vi "test_RS-xxx Write.vi"(8 "error in (no error)":errorcluster, 11 "TestCase in":refnum<class "Instrument Addon Serial Protocols Unit Tests.lvclass">) -> (0 "error out":errorcluster, 3 "TestCase out":refnum<class "Instrument Addon Serial Protocols Unit Tests.lvclass">)   [LabVIEW 2018, in "Instrument Addon Serial Protocols Unit Tests.lvclass"]
uses:
  Instrument Addon Serial Protocols Unit Tests.lvclass
  Listener/Listener.lvclass
  Listener/ListenerClassControls/Operation.ctl
  RS-xxx/RS-xxx.lvclass
  C:/Dev/niveristand-instrument-addon-classes/Source/Protocols/Protocol Parent/Protocol Parent.lvclass
  <vilib>/Platform/TimedLoop/XDataNode/timing_clust.ctl
  <vilib>/Platform/TimedLoop/XDataNode/nitl_modes.ctl
  <vilib>/Platform/TimedLoop/XDataNode/wakeup.ctl
  RS-xxx/RS-xxx.lvclass/RS-xxx.ctl
  <vilib>/platform/TimedLoop/XDataNode/XDataNode.xnode
  <vilib>/addons/_JKI Toolkits/VI Tester/TestCase.llb/TestCase.lvclass
  <vilib>/Platform/TimedLoop/XDataNode/XDNodeRunTimeDep.lvlib
  C:/Program Files (x86)/National Instruments/LabVIEW 2018/vi.lib/addons/_JKI Toolkits/VI Tester/TestCase.llb/TestCase.lvclass
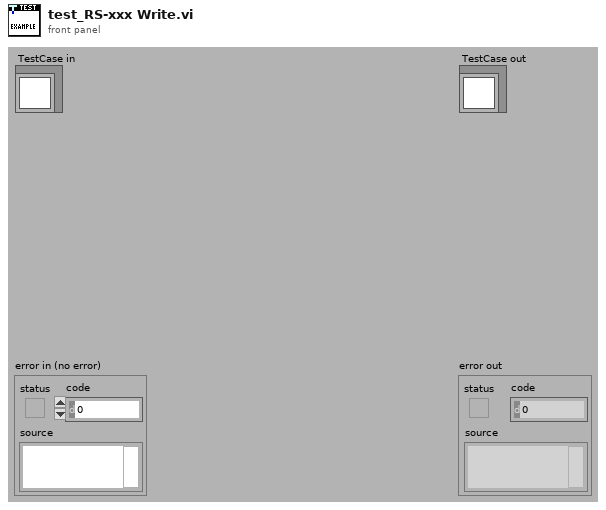
[diagram p1: front panel]
types:
  T1 = typedef "Listener.lvclass/Operation.ctl" = enum16{"Read", "Write"}
  T2 = typedef "XDNodeRunTimeDep.lvlib/timing_clust.ctl" = cluster{"Expected End [f-1]":u64, "Actual End [f-1]":u64, "Finished Late? [f-1]":bool, "Expected End [i-1]":u64, "Actual End [i-1]":u64, "Finished Late? [i-1]":bool, "Expected Start [i]":u64, "Actual Start [i]":u64, "Expected Start [f]":u64, "Actual Start [f]":u64, "Source Name":string, "Structure Name":string, "Period":i64, "Deadline":i64, "Offset":i64, "Start":i64, "Priority":i32, "Timeout":i32, "Mode":T3, "Wakeup Reason":T4, "Error":errorcluster, "Source Type":string, "Secondary Source Type":string, "Global End Time":u64, "Global Start Time":u64, "Frame Duration":u64, "Iteration Duration":u64, "Assigned CPU":i32, "I/O Scan Engine Mode":u32}
  T3 = typedef "XDNodeRunTimeDep.lvlib/nitl_modes.ctl" = enum32{"No Change", "Process missed periods, maintain original phase", "Discard missed periods, maintain original phase", "Process missed periods, ignore original phase", "Discard missed periods, ignore original phase"}
  T4 = typedef "XDNodeRunTimeDep.lvlib/wakeup.ctl" = enum32{"Normal", "Aborted", "Asynchronous wakeup", "Timing source error", "Timed loop error", "Timeout"}
  T5 = typedef "Listener.lvclass/RS-xxx Data Structure.ctl" = cluster{"Virtual COM Port Settings 1":cluster{"Port":string, "Baud Rate":u32, "Data Bits":u16, "Parity":enum16{"None", "Odd", "Even", "Mark", "Space"}, "Stop Bits":u16, "Flow Control":u16, "XON":enum16{"NUL", "SOH", "STX", "ETX", "EOT", "ENQ", "ACK", "BEL", "BS", "HT", "LF", "VT", "FF", "CR", "SO", "SI", "DLE", "DC1", "DC2", "DC3", "DC4", "NAK", "SYN", "ETB", "CAN", "EM", "SUB", "ESC", "FS", "GS", "RS", "US", "SP", "!", "\"", "#", "$", "%", "&", "'", "(", ")", "*", "+", ",", "- (-)", ".", "/", "0", "1", "2", "3", "4", "5", "6", "7", "8", "9", ":", ";", "<", "=", ">", "?", "@", "A", "B", "C", "D", "E", "F", "G", "H", "I", "J", "K", "L", "M", "N", "O", "P", "Q", "R", "S", "T", "U", "V", "W", "X", "Y", "Z", "[", "\\", "]", "^", "_", "`", "a", "b", "c", "d", "e", "f", "g", "h", "i", "j", "k", "l", "m", "n", "o", "p", "q", "r", "s", "t", "u", "v", "w", "x", "y", "z", "{", "|", "}", "~"}, "XOFF":enum16{"NUL", "SOH", "STX", "ETX", "EOT", "ENQ", "ACK", "BEL", "BS", "HT", "LF", "VT", "FF", "CR", "SO", "SI", "DLE", "DC1", "DC2", "DC3", "DC4", "NAK", "SYN", "ETB", "CAN", "EM", "SUB", "ESC", "FS", "GS", "RS", "US", "SP", "!", "\"", "#", "$", "%", "&", "'", "(", ")", "*", "+", ",", "- (-)", ".", "/", "0", "1", "2", "3", "4", "5", "6", "7", "8", "9", ":", ";", "<", "=", ">", "?", "@", "A", "B", "C", "D", "E", "F", "G", "H", "I", "J", "K", "L", "M", "N", "O", "P", "Q", "R", "S", "T", "U", "V", "W", "X", "Y", "Z", "[", "\\", "]", "^", "_", "`", "a", "b", "c", "d", "e", "f", "g", "h", "i", "j", "k", "l", "m", "n", "o", "p", "q", "r", "s", "t", "u", "v", "w", "x", "y", "z", "{", "|", "}", "~"}, "End Read on Termination Character":bool, "End Write on Termination Character":bool, "Termination Character":u8}, "Virtual COM Port Settings 2":cluster{"Port":string, "Baud Rate":u32, "Data Bits":u16, "Parity":enum16{"None", "Odd", "Even", "Mark", "Space"}, "Stop Bits":u16, "Flow Control":u16, "XON":enum16{"NUL", "SOH", "STX", "ETX", "EOT", "ENQ", "ACK", "BEL", "BS", "HT", "LF", "VT", "FF", "CR", "SO", "SI", "DLE", "DC1", "DC2", "DC3", "DC4", "NAK", "SYN", "ETB", "CAN", "EM", "SUB", "ESC", "FS", "GS", "RS", "US", "SP", "!", "\"", "#", "$", "%", "&", "'", "(", ")", "*", "+", ",", "- (-)", ".", "/", "0", "1", "2", "3", "4", "5", "6", "7", "8", "9", ":", ";", "<", "=", ">", "?", "@", "A", "B", "C", "D", "E", "F", "G", "H", "I", "J", "K", "L", "M", "N", "O", "P", "Q", "R", "S", "T", "U", "V", "W", "X", "Y", "Z", "[", "\\", "]", "^", "_", "`", "a", "b", "c", "d", "e", "f", "g", "h", "i", "j", "k", "l", "m", "n", "o", "p", "q", "r", "s", "t", "u", "v", "w", "x", "y", "z", "{", "|", "}", "~"}, "XOFF":enum16{"NUL", "SOH", "STX", "ETX", "EOT", "ENQ", "ACK", "BEL", "BS", "HT", "LF", "VT", "FF", "CR", "SO", "SI", "DLE", "DC1", "DC2", "DC3", "DC4", "NAK", "SYN", "ETB", "CAN", "EM", "SUB", "ESC", "FS", "GS", "RS", "US", "SP", "!", "\"", "#", "$", "%", "&", "'", "(", ")", "*", "+", ",", "- (-)", ".", "/", "0", "1", "2", "3", "4", "5", "6", "7", "8", "9", ":", ";", "<", "=", ">", "?", "@", "A", "B", "C", "D", "E", "F", "G", "H", "I", "J", "K", "L", "M", "N", "O", "P", "Q", "R", "S", "T", "U", "V", "W", "X", "Y", "Z", "[", "\\", "]", "^", "_", "`", "a", "b", "c", "d", "e", "f", "g", "h", "i", "j", "k", "l", "m", "n", "o", "p", "q", "r", "s", "t", "u", "v", "w", "x", "y", "z", "{", "|", "}", "~"}, "End Read on Termination Character":bool, "End Write on Termination Character":bool, "Termination Character":u8}, "Data":string, "Data Length":u32}
  T6 = cluster{"Port":string, "Baud Rate":u32, "Data Bits":u16, "Parity":enum16{"None", "Odd", "Even", "Mark", "Space"}, "Stop Bits":u16, "Flow Control":u16, "XON":enum16{"NUL", "SOH", "STX", "ETX", "EOT", "ENQ", "ACK", "BEL", "BS", "HT", "LF", "VT", "FF", "CR", "SO", "SI", "DLE", "DC1", "DC2", "DC3", "DC4", "NAK", "SYN", "ETB", "CAN", "EM", "SUB", "ESC", "FS", "GS", "RS", "US", "SP", "!", "\"", "#", "$", "%", "&", "'", "(", ")", "*", "+", ",", "- (-)", ".", "/", "0", "1", "2", "3", "4", "5", "6", "7", "8", "9", ":", ";", "<", "=", ">", "?", "@", "A", "B", "C", "D", "E", "F", "G", "H", "I", "J", "K", "L", "M", "N", "O", "P", "Q", "R", "S", "T", "U", "V", "W", "X", "Y", "Z", "[", "\\", "]", "^", "_", "`", "a", "b", "c", "d", "e", "f", "g", "h", "i", "j", "k", "l", "m", "n", "o", "p", "q", "r", "s", "t", "u", "v", "w", "x", "y", "z", "{", "|", "}", "~"}, "XOFF":enum16{"NUL", "SOH", "STX", "ETX", "EOT", "ENQ", "ACK", "BEL", "BS", "HT", "LF", "VT", "FF", "CR", "SO", "SI", "DLE", "DC1", "DC2", "DC3", "DC4", "NAK", "SYN", "ETB", "CAN", "EM", "SUB", "ESC", "FS", "GS", "RS", "US", "SP", "!", "\"", "#", "$", "%", "&", "'", "(", ")", "*", "+", ",", "- (-)", ".", "/", "0", "1", "2", "3", "4", "5", "6", "7", "8", "9", ":", ";", "<", "=", ">", "?", "@", "A", "B", "C", "D", "E", "F", "G", "H", "I", "J", "K", "L", "M", "N", "O", "P", "Q", "R", "S", "T", "U", "V", "W", "X", "Y", "Z", "[", "\\", "]", "^", "_", "`", "a", "b", "c", "d", "e", "f", "g", "h", "i", "j", "k", "l", "m", "n", "o", "p", "q", "r", "s", "t", "u", "v", "w", "x", "y", "z", "{", "|", "}", "~"}, "End Read on Termination Character":bool, "End Write on Termination Character":bool, "Termination Character":u8}
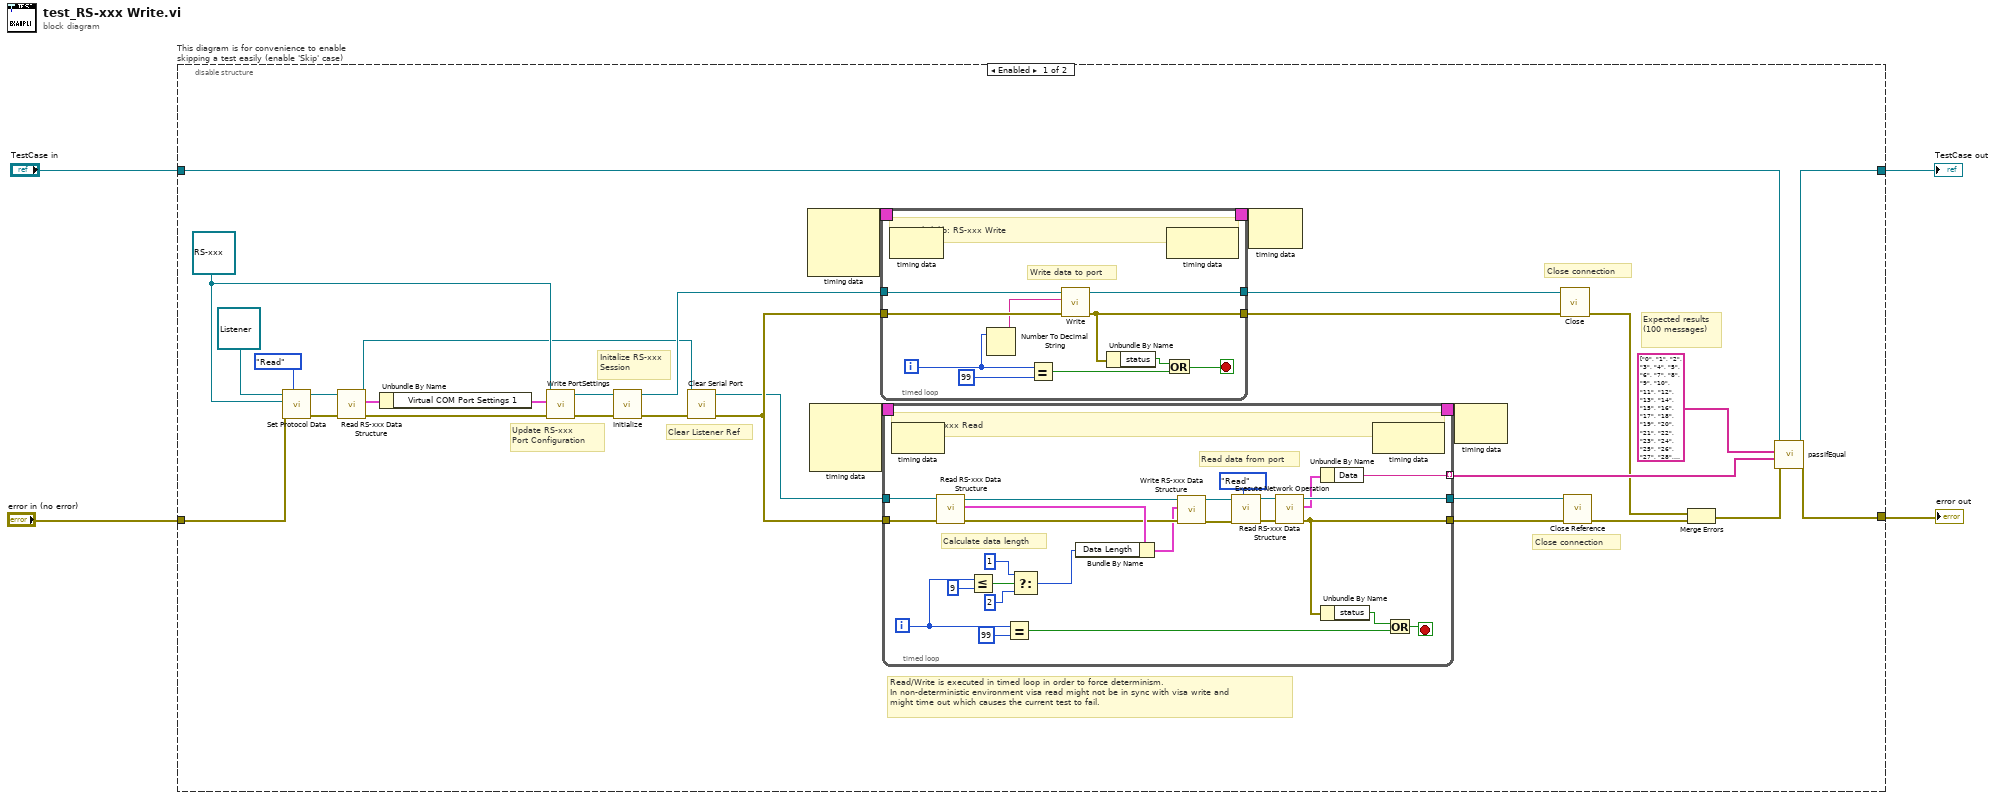
[diagram p0: block diagram]
diagram:
  n1 = disable-structure "This diagram is for convenience to enable skipping a test easily (enable 'Skip' case)" shown="Enabled" {
    disable-tunnel: "TestCase in" -> [w36 w83]
    disable-tunnel: [w35 w81] -> w1
    disable-tunnel: [w34 w82] -> w3
    disable-tunnel: "error in (no error)" -> [w33 w80]
    frame Enabled {
      w23 = refnum<class "RS-xxx.lvclass"> refnum ("Protocols.lvlib:RS-xxx.lvclass")
      # "Clear Listener Ref"
      # "Update RS-xxx \nPort Configuration"
      # "Initalize RS-xxx\nSession"
      # "Close connection"
      # "Close connection"
      # "Read/Write is executed in timed loop in order to force determinism.\nIn non-deterministic environment visa read might not be in sync with visa write and\nmight time out which causes the current test to fail."
      # "Expected results\n(100 messages)"
      n2 = call "Set Protocol Data.vi"("Operation"=Operation."Read", "error in (no error)"=w33, "Protocols.lvlib:Protocol Parent.lvclass"=w23, "Listener In.lvclass"=refnum<class "Listener.lvclass"> refnum ("Listener.lvclass")) -> ("error out"=w24:errorcluster, "Listener Out.lvclass"=w25:refnum<class "Listener.lvclass">)  [unwired: 6 in]
      n3 = call-dynamic "Read RS-xxx Data Structure.vi"("error in (no error)"=w24, "Listener in"=w25) -> ("error out"=w12:errorcluster, "RS-xxx Data Structure"=w20:T5, "Listener out"=w9:refnum<class "Listener.lvclass">)  [unwired: 7 in]
      n4 = Unbundle By Name(w20) -> ("Virtual COM Port Settings 1"=w19:T6)
      n5 = call "Write PortSettings.vi"("error in (no error)"=w12, "Cluster"=w19, "RS232 in"=w23) -> ("error out"=w13:errorcluster, "RS232 out"=w22:refnum<class "RS-xxx.lvclass">)  [unwired: 7 in]
      n6 = call-dynamic "Initialize.vi"("error in (no error)"=w13, "RS232 in"=w22) -> ("error out"=w8:errorcluster, "RS232 out"=w21:refnum<class "RS-xxx.lvclass">)  [unwired: 8 in]
      n7 = call "Clear Serial Port.vi"("error in (no error)"=w8, "Listener In.lvclass"=w9) -> ("error out"=w7:errorcluster, "Listener out"=w6:refnum<class "Listener.lvclass">)  [unwired: 8 in]
      n8 = node-c288() -> (w17:T2)  [unwired: 3 in]
      n9 = node-c288() -> (w15:T2)  [unwired: 3 in]
      n10 = timed-loop {
        tunnel: [w75] -> w27
        tunnel: w21 -> [w74]
        timing: w17 -> [_]
        timing-out: [_] -> w16
        tunnel: w7 -> [w73]
        tunnel: [w67] -> w28
        i -> [w68]
        stop <- w71 stop-if-true
        # "Write data to port"
        # "Protocols.lvlib: RS-xxx Write"
        n11 = node-c288() -> ()  [unwired: 1 in, 1 out]
        n12 = Number To Decimal String(number=w68) -> (decimal integer string=w69:string)  [unwired: 1 in]
        n13 = Equal?(x=w68, y=99) -> (x = y?=w72:bool)
        n14 = call-dynamic "Write.vi"("error in (no error)"=w73, "String"=w69, "RS232 in"=w74) -> ("error out"=w67:errorcluster, "RS232 out"=w75:refnum<class "RS-xxx.lvclass">)  [unwired: 7 in]
        n15 = Unbundle By Name(w67) -> ("status"=w66:bool)
        n16 = Or(x=w66, y=w72) -> (x .or. y?=w71:bool)
        n17 = node-c288() -> ()  [unwired: 1 in, 1 out]
      }
      n18 = timed-loop {
        tunnel: [w61] -> w11
        tunnel: [w56] -> w18 mode=indexing
        tunnel: w6 -> [w53]
        timing: w15 -> [_]
        timing-out: [_] -> w14
        tunnel: w7 -> [w52]
        tunnel: [w39] -> w26
        i -> [w49]
        stop <- w59 stop-if-true
        # "Calculate data length"
        # "Read data from port"
        # "Listener: RS-xxx Read"
        n19 = node-c288() -> ()  [unwired: 1 in, 1 out]
        n20 = call-dynamic "Read RS-xxx Data Structure.vi"("error in (no error)"=w52, "Listener in"=w53) -> ("error out"=w42:errorcluster, "RS-xxx Data Structure"=w44:T5, "Listener out"=w40:refnum<class "Listener.lvclass">)  [unwired: 7 in]
        n21 = Less Or Equal?(x=w49, y=9) -> (x <= y?=w47:bool)
        n22 = Equal?(x=w49, y=99) -> (x = y?=w54:bool)
        n23 = Select(t=u32 1 ("y"), s=w47, f=u32 2) -> (s? t:f=w43:u32)
        n24 = Bundle By Name(cluster=w44, "Data Length"=w43) -> (w41:T5)
        n25 = call-dynamic "Write RS-xxx Data Structure.vi"("error in (no error)"=w42, "RS-xxx Data Structure"=w41, "Listener in"=w40) -> ("error out"=w51:errorcluster, "Listener out"=w50:refnum<class "Listener.lvclass">)  [unwired: 7 in]
        n26 = call "Execute Network Operation.vi"("Operation"=Operation."Read", "error in (no error)"=w51, "Listener In.lvclass"=w50) -> ("error out"=w58:errorcluster, "Listener Out.lvclass"=w57:refnum<class "Listener.lvclass">)  [unwired: 7 in]
        n27 = call-dynamic "Read RS-xxx Data Structure.vi"("error in (no error)"=w58, "Listener in"=w57) -> ("error out"=w39:errorcluster, "RS-xxx Data Structure"=w37:T5, "Listener out"=w61:refnum<class "Listener.lvclass">)  [unwired: 7 in]
        n28 = Unbundle By Name(w37) -> ("Data"=w56:string)
        n29 = Unbundle By Name(w39) -> ("status"=w38:bool)
        n30 = node-c288() -> ()  [unwired: 1 in, 1 out]
        n31 = Or(x=w38, y=w54) -> (x .or. y?=w59:bool)
      }
      n32 = node-c288(w16) -> ()  [unwired: 1 out]
      n33 = node-c288(w14) -> ()  [unwired: 1 out]
      n34 = call-dynamic "Close.vi"("error in (no error)"=w28, "RS232 in"=w27) -> ("error out"=w10:errorcluster)  [unwired: 8 in, 1 out]
      n35 = call "Close Reference.vi"("error in (no error)"=w26, "Listener In.lvclass"=w11) -> ("error out"=w29:errorcluster)  [unwired: 8 in, 1 out]
      n36 = Merge Errors(w10, w29) -> (w30:errorcluster)
      n37 = call-dynamic "passIfEqual.vi"("error in (no error)"=w30, "y"=w18, "x"=string[] ["0", "1", "2", "3", "4", "5", "6", "7", "8", "9", "10", "11", "12", "13", "14", "15", "16", "17", "18", "19", "20", "21", "22", "23", "24", "25", "26", "27", "28", "29", "30", "31", "32", "33", "34", "35", "36", "37", "38", "39", "40", "41", "42", "43", "44", "45", "46", "47", "48", "49", "50", "51", "52", "53", "54", "55", "56", "57", "58", "59", "60", "61", "62", "63", "64", "65", "66", "67", "68", "69", "70", "71", "72", "73", "74", "75", "76", "77", "78", "79", "80", "81", "82", "83", "84", "85", "86", "87", "88", "89", "90", "91", "92", "93", "94", "95", "96", "97", "98", "99"] ("Array"), "TestCase in"=w36) -> ("error out"=w34:errorcluster, "TestCase out"=w35:refnum<class "Instrument Addon Serial Protocols Unit Tests.lvclass">)  [unwired: 6 in]
    }
    frame Disabled {
      # "skip test result while test is under development"
      n38 = call <vilib>:"skip.vi"("error in (no error)"=w80, "TestCase in"=w83) -> ("error out"=w82:errorcluster, "TestCase out"=w81:refnum<class "Instrument Addon Serial Protocols Unit Tests.lvclass">)  [unwired: 8 in]
    }
  }
  "error out" <- w3
  "TestCase out" <- w1
